vi "数据储存-D-shunt.vi"(8 "错误输入":errorcluster, 10 "2D data":dbl[][](array[numeric]) caption="二维数据", 11 "数据储存":string) -> (0 "error out":errorcluster caption="错误输出")   [LabVIEW 2021]
uses:
  <vilib>/Utility/file.llb/Write Delimited Spreadsheet (DBL).vi
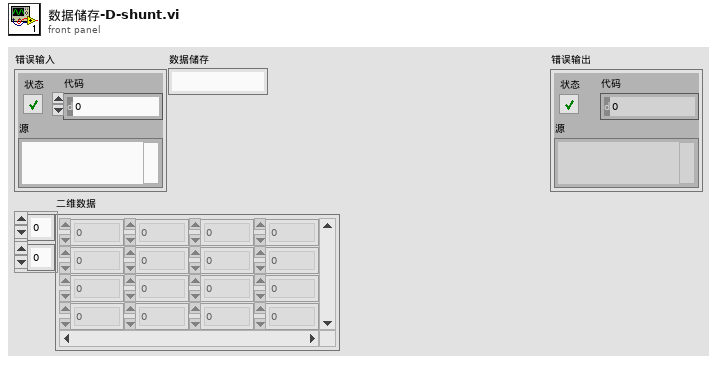
[diagram p1: front panel]
types:
  T1 = enum16{"open", "replace", "create", "open or create", "replace or create", "replace or create with confirmation"}
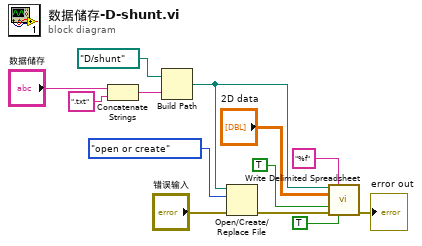
[diagram p0: block diagram]
diagram:
  n1 = Concatenate Strings("数据储存", ".txt") -> (w3:string)
  n2 = Build Path(base path=path "D:/shunt" ("file path (dialog if empty)"), name or relative path=w3) -> (appended path=w11:path)
  n3 = Open/Create/Replace File(file path (use dialog)=w11, error in="错误输入", operation (0:open)=T1."open or create" ("操作(0:open)")) -> (error out=w7:errorcluster)  [unwired: 3 in, 2 out]
  n4 = call-poly <vilib>:"Write Delimited Spreadsheet.vi"("file path (dialog if empty)"=w11, "format (%.3f)"="%f", "2D data"="2D data", "append to file? (new file:F)"=TRUE, "error in (no error)"=w7, "transpose? (no:F)"=TRUE) -> ("error out"=→"error out":errorcluster)  [unwired: 8 in, 1 out]
